vi "SetColumnHeaders.vi"(8 "error in (no error)":errorcluster, 10 "column headers":string[](array[string]), 11 "Excel refnum":T1) -> (0 "error out":errorcluster, 3 "Excel refnum out":T1)   [LabVIEW 2020, in "NI_ExcelFile.lvlib"]
doc: "Sets the header for every column in a .xlsx file.\n \nExcel refnum: Specifies a reference to the .xlsx file on which to perform the operation. Use the Create VI to create or open the refnum.\n\ncolumn headers: Specifies the header for every column in the .xlsx file. If you do not set the header for the columns, this VI automatically creates headers for each column using the following format: \"Untitled i\", where i is an integer.\n\nerror in: describes error conditions that occur before this node runs. This input provides standard error in functionality.\n\nExcel refnum out: Returns a Microsoft Excel file reference to the .xlsx file on which you performed the operation.\n\nerror out: contains error information. This output provides standard error out functionality."
uses:
  <vilib>/express/express shared/NI_ExcelFile/NI_ExcelFile.lvlib
  <vilib>/express/express shared/NI_ExcelFile/Ctrls/ExcelRefnum.ctl
  <vilib>/express/express shared/NI_ExcelFile/Ctrls/MainData.ctl
  <vilib>/express/express shared/NI_ExcelFile/Ctrls/StreamMode.ctl
  <vilib>/express/express shared/NI_ExcelFile/Ctrls/TimeColumnMode.ctl
  <vilib>/express/express shared/NI_ExcelFile/Ctrls/FileAttribute.ctl
  <vilib>/express/express shared/NI_ExcelFile/Ctrls/Columns.ctl
  <vilib>/express/express shared/NI_ExcelFile/Ctrls/ColumnInfo.ctl
  <vilib>/express/express shared/NI_ExcelFile/Ctrls/DataType.ctl
  <vilib>/express/express shared/NI_ExcelFile/Ctrls/wd_recordInfo.ctl
  <vilib>/express/express shared/NI_ExcelFile/Ctrls/disk_TemplateFile.ctl
  <vilib>/express/express shared/NI_ExcelFile/Ctrls/meta_file.ctl
  <vilib>/express/express shared/NI_ExcelFile/Ctrls/meta_Block.ctl
  <vilib>/express/express shared/NI_ExcelFile/Ctrls/meta_BlockType.ctl
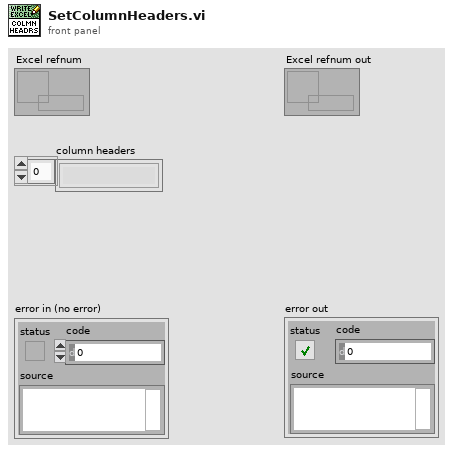
[diagram p1: front panel]
types:
  T1 = typedef "NI_ExcelFile.lvlib/ExcelRefnum.ctl" = refnum<data-value>
  T2 = typedef "NI_ExcelFile.lvlib/MainData.ctl" = cluster{"TargetFile":path, "StreamMode":T3, "Append?":bool, "ChunkSize":u64, "TimeColumnMode":T4, "TimestampFormat":string, "AbsoluteTime?":bool, "FileAttribute ":T5, "Column":T6, "FileRef":refnum<k1>, "MemoryRef":refnum<data-value>[], "RecordInfo":T9[], " ChannelPreviousInfo":u32[], "ChannelFirstRecord":u32[], "PredefinedFormattedValueLength":i64, "DiskTemplate":T10}
  T3 = typedef "NI_ExcelFile.lvlib/StreamMode.ctl" = enum16{"File", "Memory"}
  T4 = typedef "NI_ExcelFile.lvlib/TimeColumnMode.ctl" = enum16{"Empty", "OnePerCh", "One"}
  T5 = typedef "NI_ExcelFile.lvlib/FileAttribute.ctl" = cluster{"Creator":string, "Title":string, "SheetName":string}
  T6 = typedef "NI_ExcelFile.lvlib/Columns.ctl" = T7[]
  T7 = typedef "NI_ExcelFile.lvlib/ColumnInfo.ctl" = cluster{"Header":string, "Format":string, "DataType":T8, "Length":u64}
  T8 = typedef "NI_ExcelFile.lvlib/DataType.ctl" = enum16{"DDT", "WFM", "Array of STR", "Array of DBL", "Array of I8", "Array of I16", "Array of I32", "Array of I64", "Array of SGL", "Array of U8", "Array of U16", "Array of U32", "Array of U64", "Array of Time"}
  T9 = typedef "NI_ExcelFile.lvlib/wd_recordInfo.ctl" = cluster{"ChannelIndex":u32, "StartIndex":u64, "Length":u64, "Previous":i32, "Next":i32}
  T10 = typedef "NI_ExcelFile.lvlib/disk_TemplateFile.ctl" = cluster{"XMLRef":refnum<file>[], "ZipPath":path, "MetaFile":T11, "TempFolder":path}
  T11 = typedef "NI_ExcelFile.lvlib/meta_file.ctl" = cluster{"Ref":refnum<file>, "NextRow":i32, "NextPosition":i64, "Block":T12[]}
  T12 = typedef "NI_ExcelFile.lvlib/meta_Block.ctl" = cluster{"Version":u16, "Type":T13, "Length":i32, "Data":string}
  T13 = typedef "NI_ExcelFile.lvlib/meta_BlockType.ctl" = enum16{"NITag", "File", "Column"}
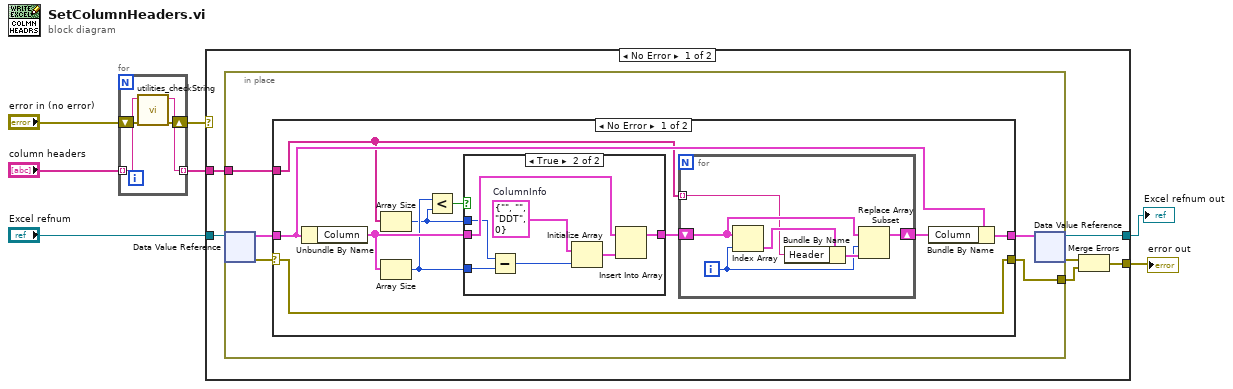
[diagram p0: block diagram]
diagram:
  n1 = for {
    tunnel: "column headers" -> [w11] mode=indexing
    shift-right: [w9] -> w3
    shift-left: "error in (no error)" -> [w10]
    tunnel: [w8] -> w1 mode=indexing
    n2 = call <vilib>:"utilities_checkString.vi"("error in (no error)"=w10, "String"=w11) -> ("error out"=w9:errorcluster, "String out"=w8:string)  [unwired: 8 in]
  }
  n3 = case shown="No Error" w3 {
    selector: w3 -> [_ w50]
    tunnel: [w14 w50] -> w7
    tunnel: [w16 w49] -> w5
    tunnel: "Excel refnum" -> [w17 w49]
    tunnel: w1 -> [w12 _]
    frame No Error {
      n4 = in-place {
        in-place-border: w12 -> [w22]
        in-place-border: [w18] -> w13
        n5 = in-place-dvr #1(w17) -> (w21:T2, w19:errorcluster)
        n6 = case shown="No Error" w19 {
          selector: w19 -> [w23 w47]
          tunnel: w22 -> [w24 _]
          tunnel: w21 -> [w31 w48]
          tunnel: [w30 w48] -> w20
          tunnel: [w23 w47] -> w18
          frame No Error {
            n7 = Unbundle By Name(w31) -> ("Column"=w32:T6)
            n8 = Array Size(array=w24) -> (size(s)=w27:i32)
            n9 = Array Size(array=w32) -> (size(s)=w29:i32)
            n10 = Less?(x=w29, y=w27) -> (x < y?=w28:bool)
            n11 = case shown="True" w28 {
              tunnel: w32 -> [w39 w45]
              tunnel: w29 -> [_ w40]
              tunnel: w27 -> [_ w41]
              tunnel: [w39 w42] -> w26
              frame False {
              }
              frame True {
                w43 = T7 {"Header"="", "Format"="", "DataType"=enum."DDT", "Length"=0}  # ColumnInfo
                n12 = Subtract(x=w41, y=w40) -> (x-y=w46:i32)
                n13 = Initialize Array(w43, w46) -> (w44:T7[])
                n14 = Insert Into Array(array=w45, new element=w44) -> (w42:T6)  [unwired: 1 in]
              }
            }
            n15 = for {
              shift-right: [w38] -> w25
              shift-left: w26 -> [w34]
              tunnel: w24 -> [w33] mode=indexing
              i -> [w36]
              n16 = Index Array(array=w34, index=w36) -> (element=w35:T7)
              n17 = Bundle By Name(cluster=w35, "Header"=w33) -> (w37:T7)
              n18 = Replace Array Subset(array=w34, new element=w37, index=w36) -> (w38:T6)
            }
            n19 = Bundle By Name(cluster=w31, "Column"=w25) -> (w30:T2)
          }
          frame Error {
          }
        }
        n20 = in-place-dvr #1(w20) -> (w16:T1, w15:errorcluster)
      }
      n21 = Merge Errors(w15, w13) -> (w14:errorcluster)
    }
    frame Error {
    }
  }
  "Excel refnum out" <- w5
  "error out" <- w7
